vi "text handling.vi"() -> ()   [LabVIEW 2012]
panel:
  out "text 2":string
  in  "text":string
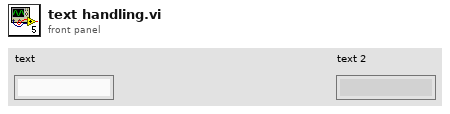
[diagram p1: front panel]
types:
  T1 = enum16{"open", "replace", "create", "open or create", "replace or create", "replace or create with confirmation"}
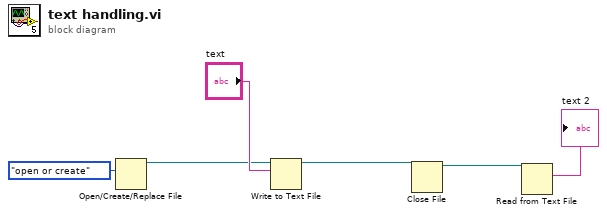
[diagram p0: block diagram]
diagram:
  n1 = Open/Create/Replace File(operation (0:open)=T1."open or create") -> (refnum out=w5:refnum<file>)  [unwired: 5 in, 2 out]
  n2 = Write to Text File(file (use dialog)=w5, text="text") -> (refnum out=w4:refnum<file>)  [unwired: 2 in, 2 out]
  n3 = Close File(refnum=w4) -> (path=w3:path)  [unwired: 1 in, 1 out]
  n4 = Read from Text File(file (use dialog)=w3) -> (text=→"text 2":string)  [unwired: 3 in, 3 out]
